vi "POISelection.vi"(5 "InvertSelection":bool, 7 "SelectAll":bool, 11 "POISelectArrayIn":cluster{"System Array":i32[], "Boolean":bool}[](array[cluster])) -> (2 "POI array":dbl[][](array[numeric]), 3 "POISelectArrayOut":cluster{"System Array":i32[], "Boolean":bool}[](array[cluster]))   [LabVIEW 2017]
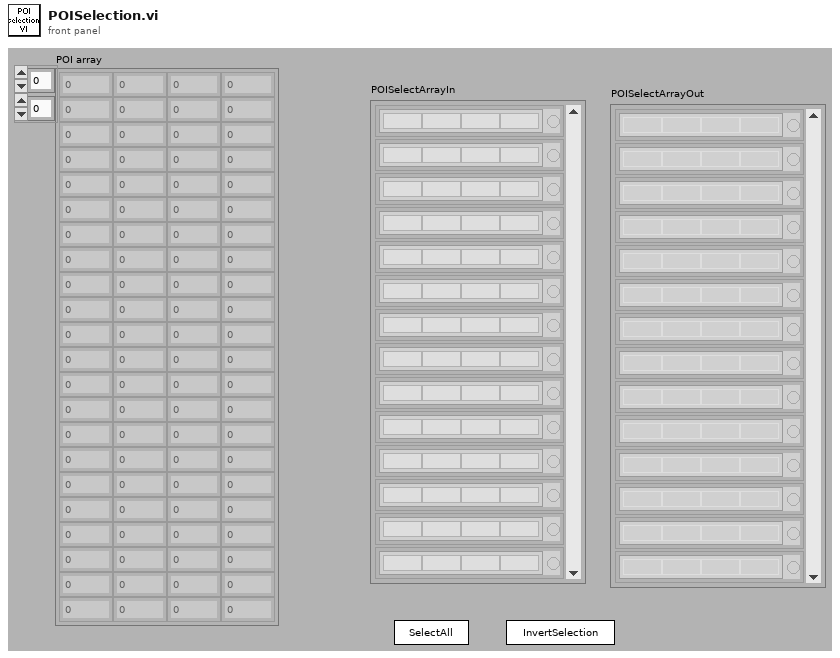
[diagram p1: front panel]
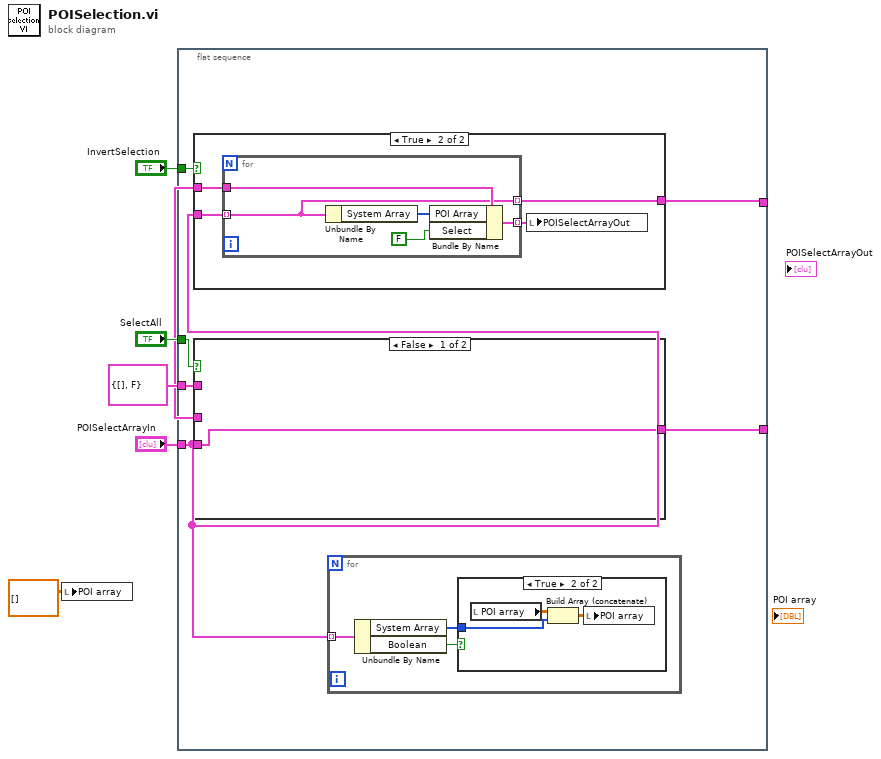
[diagram p0: block diagram]
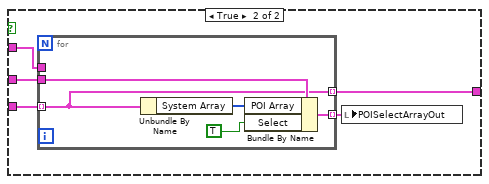
[diagram p4: hidden frame]
diagram:
  n1 = local write "POI array"(dbl[][] [] ("POI array")) -> ()
  n2 = flat-sequence {
    tunnel: "SelectAll" -> [w11]
    tunnel: "InvertSelection" -> [w10]
    tunnel: cluster{"POI Array":i32[], "Select":bool} {"POI Array"=[], "Select"=FALSE} ("System Cluster") -> [w9]
    tunnel: "POISelectArrayIn" -> [w8]
    tunnel: [w7] -> _
    tunnel: [w6] -> _
    frame #0 {
      n3 = case shown="True" w10 {
        tunnel: w9 -> [_ w20]
        tunnel: w8 -> [w18 w21]
        tunnel: [w18 w19] -> w6
        frame False {
        }
        frame True {
          n4 = for {
            tunnel: [w27] -> w22 mode=indexing
            tunnel: w21 -> [w23] mode=indexing
            tunnel: w20 -> [w25]
            tunnel: [w23] -> w19 mode=indexing
            n5 = Unbundle By Name(w23) -> ("System Array"=w24:i32[])
            n6 = Bundle By Name(cluster=w25, "POI Array"=w24, "Select"=FALSE) -> (w27:cluster{"POI Array":i32[], "Select":bool})
          }
          n7 = local write "POISelectArrayOut"(w22) -> ()
        }
      }
      n8 = case shown="False" w11 {
        tunnel: w9 -> [_ w33]
        tunnel: w8 -> [w28 w31]
        tunnel: w9 -> [_ w30]
        tunnel: [w28 w29] -> w7
        frame False {
        }
        frame True {
          n9 = for {
            tunnel: w33 -> [_]
            tunnel: [w38] -> w32 mode=indexing
            tunnel: w31 -> [w34] mode=indexing
            tunnel: w30 -> [w35]
            tunnel: [w34] -> w29 mode=indexing
            n10 = Unbundle By Name(w34) -> ("System Array"=w36:i32[])
            n11 = Bundle By Name(cluster=w35, "POI Array"=w36, "Select"=TRUE) -> (w38:cluster{"POI Array":i32[], "Select":bool})
          }
          n12 = local write "POISelectArrayOut"(w32) -> ()
        }
      }
      n13 = for {
        tunnel: w8 -> [w14] mode=indexing
        n14 = Unbundle By Name(w14) -> ("System Array"=w12:i32[], "Boolean"=w13:bool)
        n15 = case shown="True" w13 {
          tunnel: w12 -> [_ w17]
          frame False {
          }
          frame True {
            n16 = local read "POI array"() -> (w16:dbl[][])
            n17 = Build Array (concatenate)(w16, w17) -> (w15:dbl[][])
            n18 = local write "POI array"(w15) -> ()
          }
        }
      }
    }
  }
